vi "Autonomous Independent.vi"() -> ()   [LabVIEW 2013]
doc: "If AutoIDs match then TwoBall? is read from Dashboard, Else it is a control on the Front Panel\n\nINPUTS:\nTwoBall?\nState (Init)\nCollectorArmSpeed\nBrakeDistance\nSlowdownDistance\n\nSTATES:\n\nINIT: Clapper - In, SonicShifter Actuates to Low Gear, RollerPnuematic - Out, Servo - SetAngle (Indicator on Front Panel), IF TwoBall? == True: LowerArm ELSE CheckHotGoal\n\nCHECKHOTGOAL: Runs IsHotGoalDB and puts HotGoal? into Shift Register\n\nLOWERARM: Clapper - OUT, Wait = LowerArmTimeout / 2, RollerPneumatic - WAIT, Collector- LOWER\nWhen Collector has finished or after timeout from LowerArmTimeout and two other timers, Collector - STOP\nIF TwoBall? == TRUE then Collect ELSE Drive12ft\n\nPRECOLLECT: CollectorWrapper - PRECOLLECT\n\nDRIVEBACK: TankDrive -SETVALUE and DriveBackSpeed goes into both desired speeds, Wait - DriveBackWait, TankDrive - SETVALUE and 0 for both desired speeds\n\nCOLLECT: CollectWrapper - COLLECT\n\nSTOPCOLLECT: CollectWrapper - STOP\n\nLIFTARM: Collector - RAISE, Wait - LiftArmWait, Collector - STOP\n\nRAISESERVO: Servo - SETANGLE, Servo takes in RaiseServoAngle from Front Panel\n\nDRIVE12FT: Sonar - READVALUE, AutoDistance - LINEAR, Takes in Drive12ftDistance and distance from the Sonar and BrakeDistance and SlowdownDistance, TankDrive - LINEARDRIVE, Takes in both motor values from AutoDistance and MaxMotorChangeForward/Backward for Desired, TankDrive - LINEARDRIVE, Takes in 0 for Desired and MaxMotorChanges\n\nSHOOT12FT: IF not TwoBall? AND not HotGoal? then Wait - 5500 - ElapsedTime ELSE Pass, Wait - PreShootWait, ShooterWrapper - COLLECTORDOWN\n\nRAISEARM: Wait - PreRaiseArmWait, Collector - RAISE, Takes in CollectorArmSpeed, After Timeout from RaiseArmTimeout or Collector is done , Collector - STOP\n\nSHOOT3FT: Sonar - READVALUE, AutoDistance - LINEAR, Takes in Drive3ftDistance and output form Sonar and Brake/SlowdownDistance, TankDrive - SETVALUE, Takes in AutoDistance values for desired, Exits after AutoDistance is done or Drive3tfTimeout, TankDrive - SETVALUE, Takes in 0 for desired\n\nSHOOT3FT: ShooterWrapper - COLLECTORUP\n\nSTOP: Servo - SETANGLE, 0 for angle"
uses:
  AutoStates.ctl
  AutoMode.ctl
  HotGoalDetectType.ctl
  SingleSolenoidAction.ctl
  DoubleSolenoidAction.ctl
  ServoAction.ctl
  CollectorAction.ctl
  RollerAction.ctl
  TankDriveAction.ctl
  CollectorWrapAction.ctl
  SonarAction.ctl
  AutoAlignMode.ctl
  ShooterWrapperAction.ctl
  Robot Global Data.vi
panel:
  in  "PreScumbagWait":u32
  in  "HotGoalTypeDefault":T1
  out "KinectTriggered?":bool
  in  "EndInLowGear?":bool=TRUE
  in  "DriveBackWait":u32=1000
  in  "DriveBackSpeed":dbl=-1.0
  in  "PreCheckGoalWait":u32=260
  in  "BallSettleWait":u32=130
  in  "StartShootTime":u32=5000
  in  "StartInLowGear?":bool=TRUE
  in  "PreCollectWait":u32=400
  in  "AutoIDKey":i32=3061
  in  "DefaultMotorInput":dbl=1.0
  in  "DriveMinTime":u32=2000
  in  "RotateWait":u32=300
  in  "RotateMotorInput":dbl=0.7
  in  "DriveDistance":dbl=36.0 format="%#_13g"
  in  "DriveTimeout":u32=4000
  out "CheckGoalTimedOut?":bool
  in  "CheckHotGoalTimeout":u32=800
  in  "AutoDefaultMode":T2
  in  "ServoInitAngle":i32=140
  in  "RaiseServoAngle":i32=100
  in  "AccelBackward":dbl=0.1
  in  "PreRaiseArmWait":u32=500
  in  "AccelForward":dbl=0.1
  out "ElapsedTime":u32
  out "StateTime":u32
  out "CurrentState":T3
  out "RaiseArmTimedOut":bool
  out "Hot?":bool
  out "DriveTimeOut":bool
  out "LowerArmTimedOut":bool
  in  "RaiseArmTimeout":u32=800
  in  "SlowdownDistance":dbl=36.0 format="%#_13g"
  in  "BrakeDistance":dbl=12.0 format="%#_13g"
  in  "CollectorArmSpeed":dbl=1.0 format="%#_13g"
  in  "LiftArmWait":u32=200
  in  "PreDriveBackWait":u32
  in  "PreDriveBackSpeed":dbl
  in  "LowerArmTimeout":u32=800
  in  "error in":errorcluster
  out "error out":errorcluster
  # "SHOOT"
  # "SERVO"
  # "HOT GOAL"
  # "OUTPUT"
  # "ROTATE"
  # "GENERAL"
  # "DRIVE"
  # "RAISE/LOWER ARM"
  # "DEPRECATED"
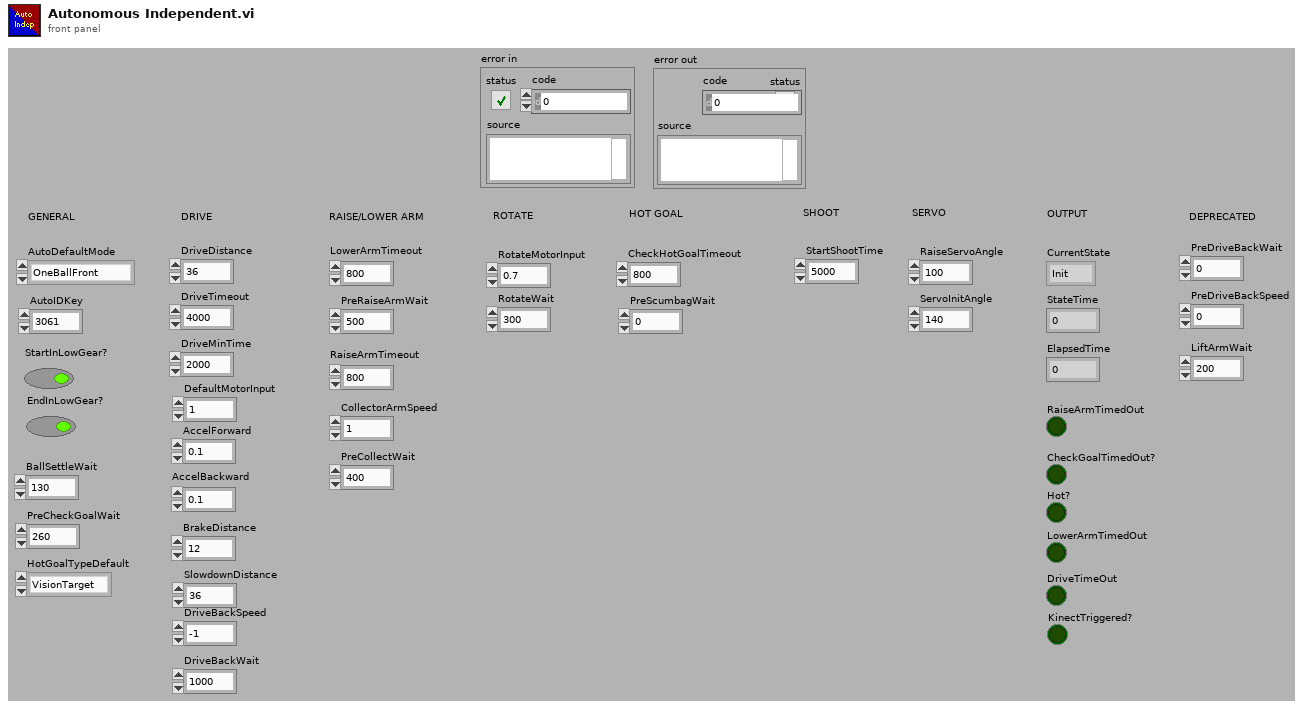
[diagram p1: front panel]
types:
  T1 = typedef "HotGoalDetectType.ctl" = enum16{"VisionTarget", "Kinect", "SoundDetect", "Webcam"}
  T2 = typedef "AutoMode.ctl" = enum16{"OneBallFront", "OneBallCollector", "TwoBallNormal", "TwoBallHot"}
  T3 = typedef "AutoStates.ctl" = enum16{"Init", "LowerArmCheckGoal", "DriveBack", "Collect", "StopCollect", "LiftArm", "RaiseServo", "Drive", "ShootCollectorUp", "RaiseArm", "ShootCollectorDown", "Rotate1", "Rotate2", "Stop"}
  T4 = typedef "SingleSolenoidAction.ctl" = enum16{"Init", "SetState", "Disable"}
  T5 = typedef "DoubleSolenoidAction.ctl" = enum16{"Init", "Middle", "In", "Out"}
  T6 = typedef "ServoAction.ctl" = enum16{"Init", "SetAngle", "GetAngle", "Lower", "Raise", "Disable"}
  T7 = typedef "CollectorAction.ctl" = enum16{"Init", "Raise", "Lower", "Stop", "GetStatus"}
  T8 = typedef "RollerAction.ctl" = enum16{"Init", "Off", "Forward", "Reverse"}
  T9 = typedef "TankDriveAction.ctl" = enum16{"Init", "LinearDrive", "SetValue", "Disable"}
  T10 = typedef "CollectorWrapAction.ctl" = enum16{"Stop", "PreCollect", "Collect"}
  T11 = typedef "AutoAlignMode.ctl" = enum16{"Fullspeed", "Linear"}
  T12 = typedef "SonarAction.ctl" = enum16{"Init", "ReadValue", "Disable"}
  T13 = typedef "ShooterWrapperAction.ctl" = enum16{"Init", "CollectorDown", "CollectorUp"}
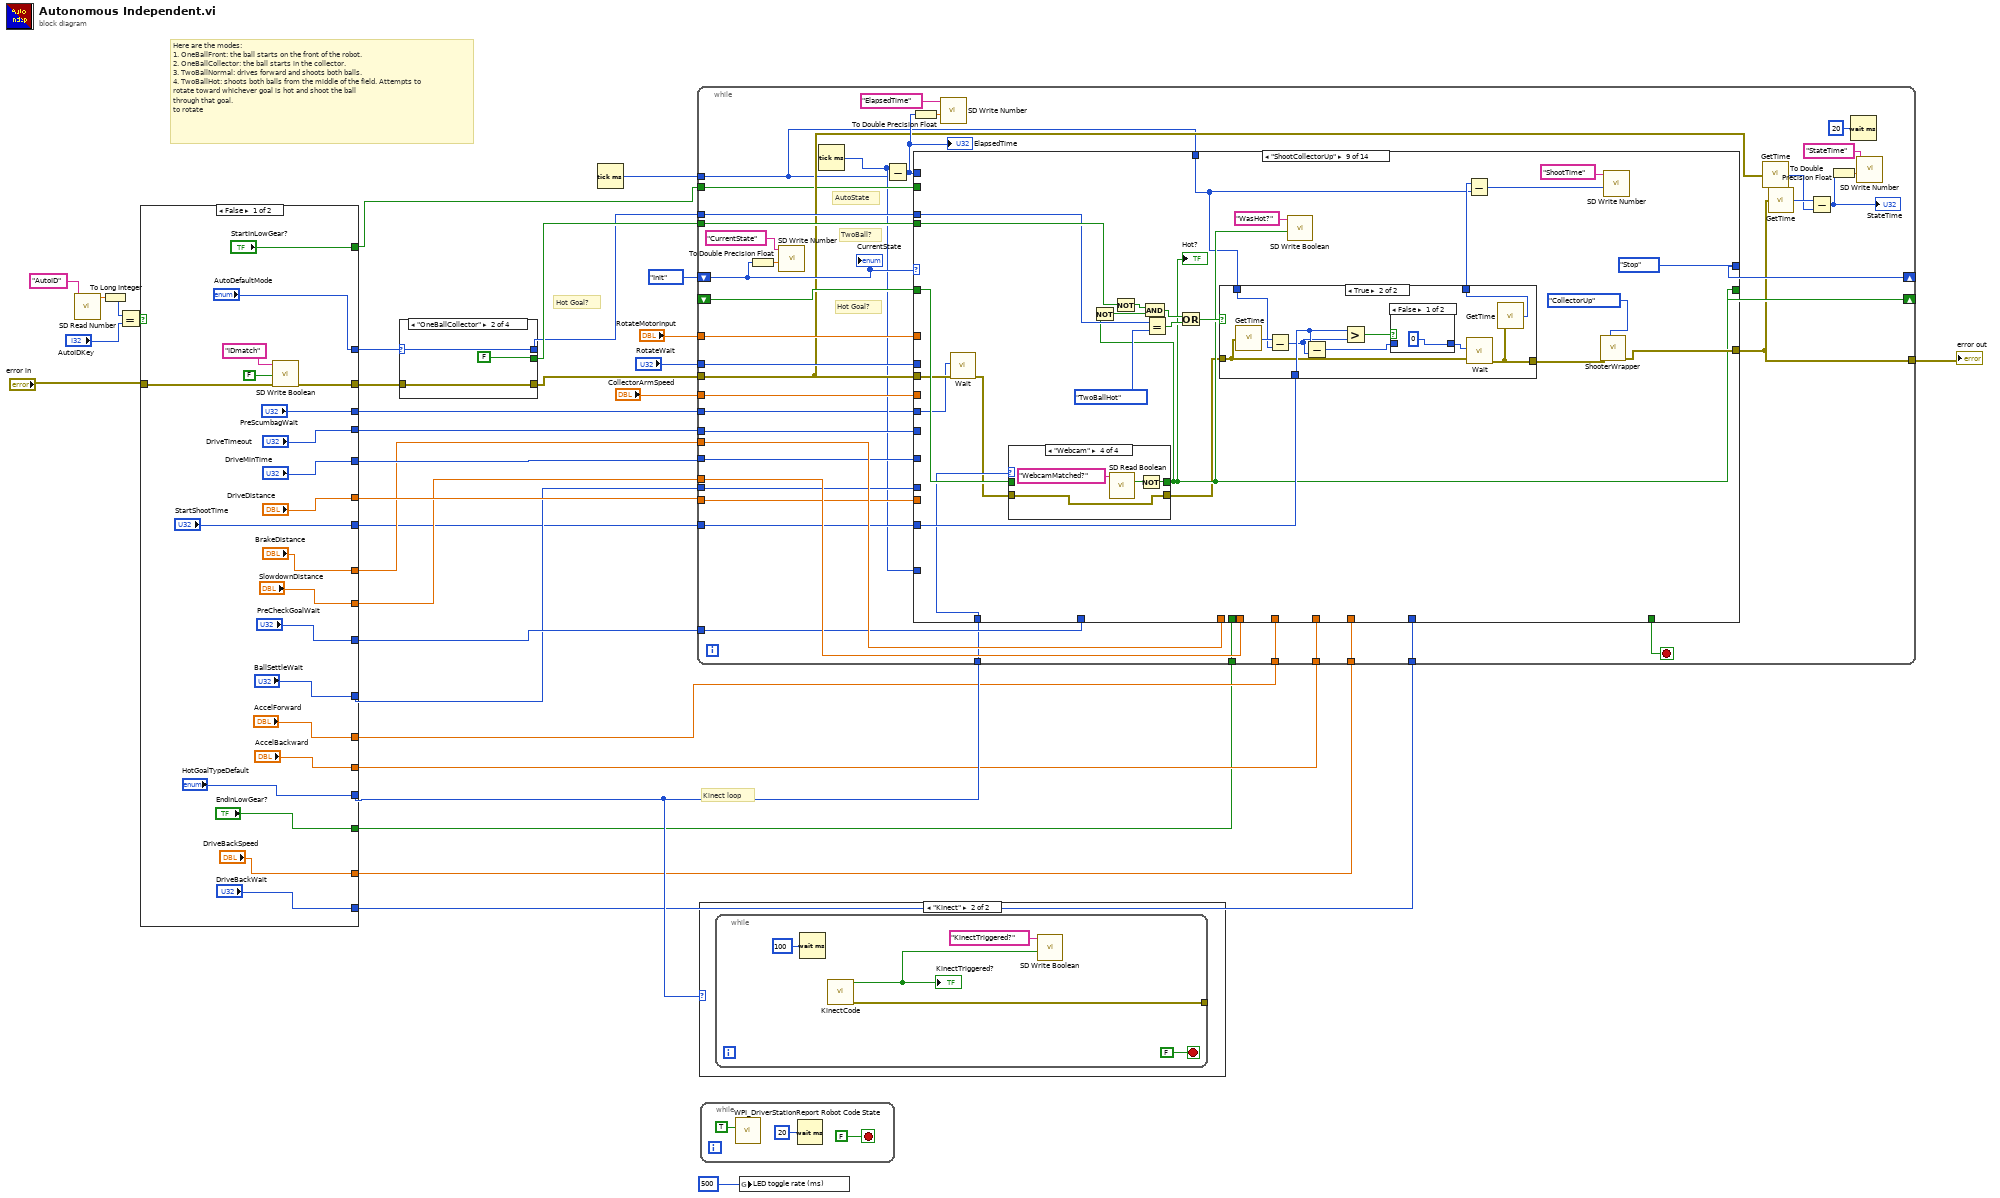
[diagram p0: block diagram]
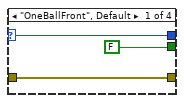
[diagram p3: hidden frame]
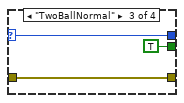
[diagram p4: hidden frame]
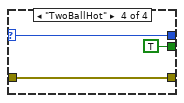
[diagram p5: hidden frame]
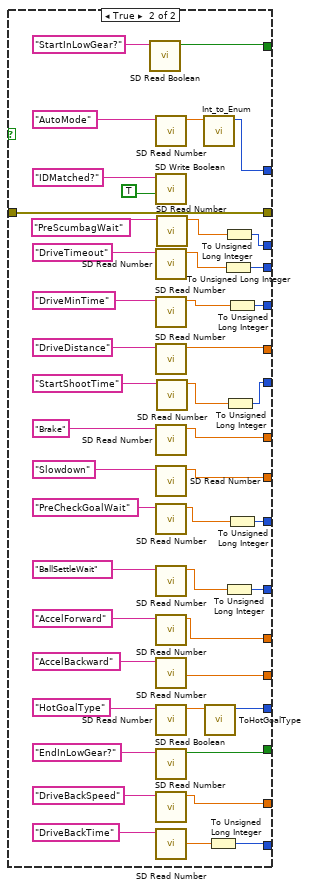
[diagram p6: hidden frame]
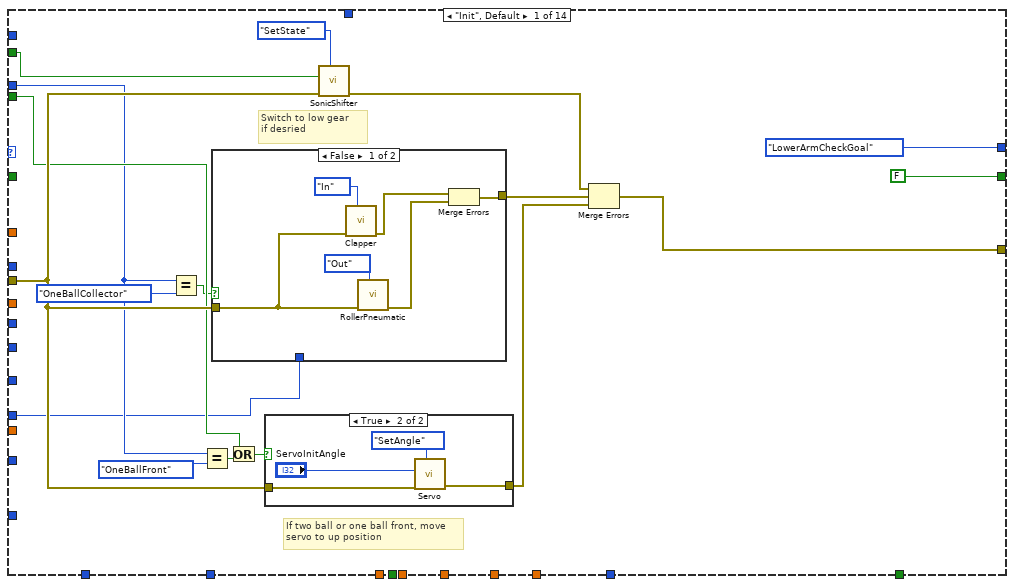
[diagram p7: hidden frame]
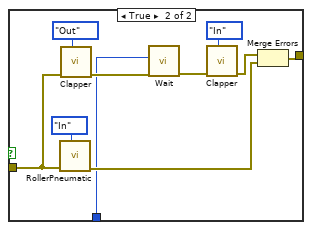
[diagram p8: hidden frame]
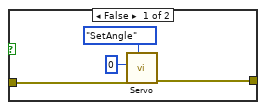
[diagram p9: hidden frame]
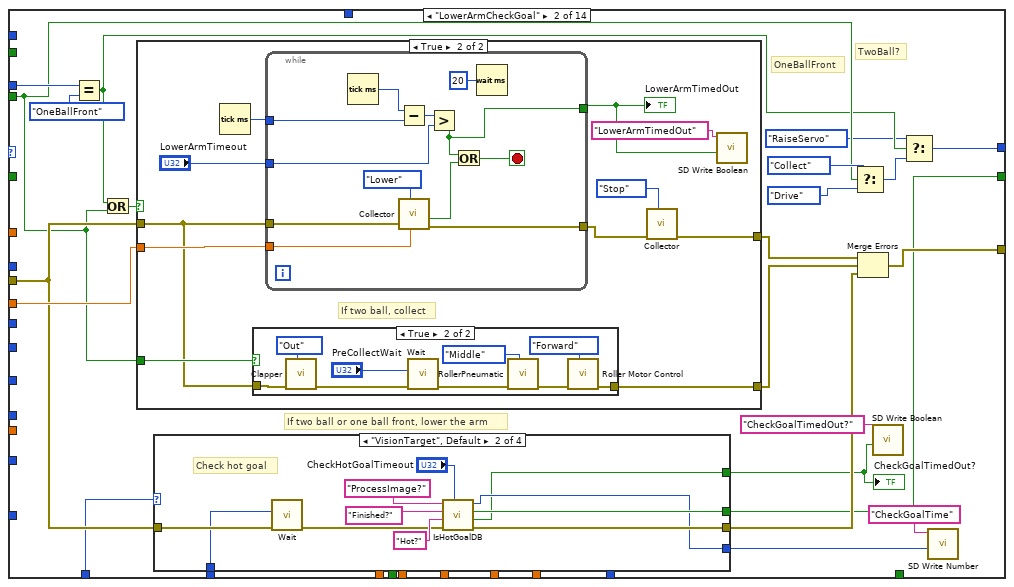
[diagram p10: hidden frame]
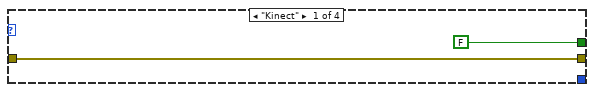
[diagram p11: hidden frame]
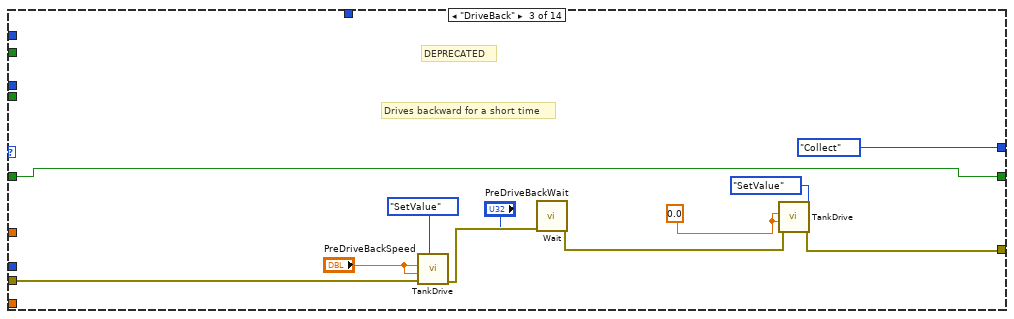
[diagram p16: hidden frame]
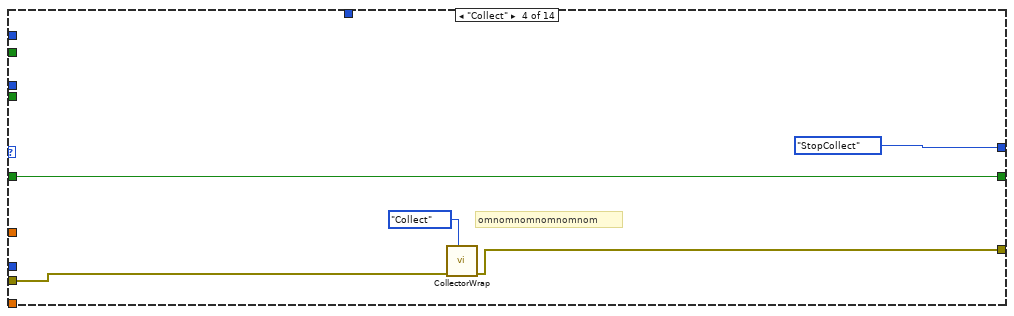
[diagram p17: hidden frame]
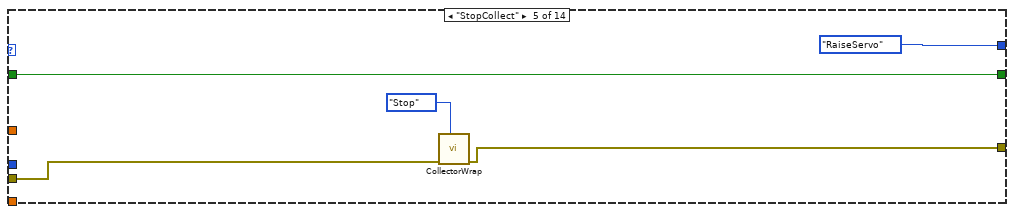
[diagram p18: hidden frame]
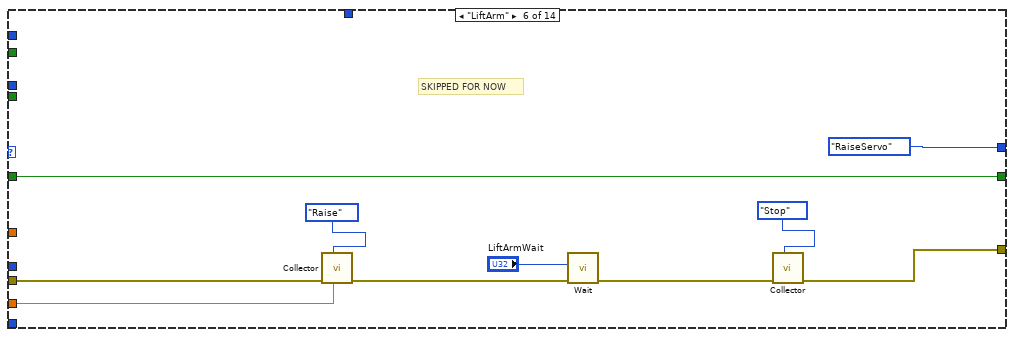
[diagram p19: hidden frame]
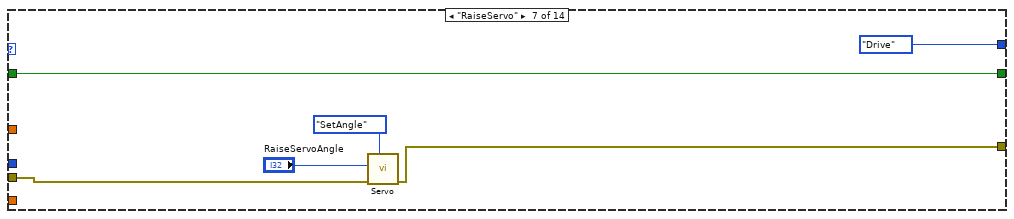
[diagram p20: hidden frame]
diagram:
  # "Kinect loop"
  # "Here are the modes:\n1. OneBallFront: the ball starts on the front of the robot.\n2. OneBallCollector: the ball starts in the collector.\n3. TwoBallNormal: drives forward and shoots both balls.\n4. TwoBallHot: shoots both balls from the middle of the field. Attempts to rotate toward whichever goal is hot and shoot the ball\nthrough that goal.\nto rotate"
  # "Hot Goal?"
  n1 = call <vilib>:"SD Read Number.vi"("Name"="AutoID") -> ("Numeric"=w33:dbl)  [unwired: 8 in, 2 out]
  n2 = To Long Integer(number=w33) -> (32bit integer=w19:i32)
  n3 = Equal?(x=w19, y="AutoIDKey") -> (x = y?=w28:bool)
  n4 = case shown="False" w28 {
    tunnel: "error in" -> [w54 w62]
    tunnel: [w53 w62] -> w24
    tunnel: ["AutoDefaultMode" w98] -> w26
    tunnel: ["DriveTimeout" w93] -> w14
    tunnel: ["DriveMinTime" w91] -> w15
    tunnel: ["DriveDistance" w89] -> w16
    tunnel: ["BrakeDistance" w87] -> w13
    tunnel: ["SlowdownDistance" w86] -> w12
    tunnel: ["PreCheckGoalWait" w83] -> w11
    tunnel: ["BallSettleWait" w80] -> w10
    tunnel: ["HotGoalTypeDefault" w76] -> w9
    tunnel: ["StartInLowGear?" w75] -> w8
    tunnel: ["AccelForward" w71] -> w7
    tunnel: ["AccelBackward" w70] -> w6
    tunnel: ["EndInLowGear?" w68] -> w5
    tunnel: ["DriveBackSpeed" w66] -> w4
    tunnel: ["DriveBackWait" w63] -> w3
    tunnel: ["StartShootTime" w59] -> w2
    tunnel: ["PreScumbagWait" w56] -> w1
    frame False {
      n5 = call <vilib>:"SD Write Boolean.vi"("error in"=w54, "Boolean"=FALSE, "Name"="IDmatch") -> ("error out"=w53:errorcluster)  [unwired: 7 in, 1 out]
    }
    frame True {
      n6 = call <vilib>:"SD Read Boolean.vi"("Name"="StartInLowGear?") -> ("Boolean"=w75:bool)  [unwired: 8 in, 2 out]
      n7 = call <vilib>:"SD Read Number.vi"("Name"="AutoMode") -> ("Numeric"=w99:dbl)  [unwired: 8 in, 2 out]
      n8 = call <vilib>:"SD Write Boolean.vi"("Boolean"=TRUE, "Name"="IDMatched?") -> ()  [unwired: 8 in, 2 out]
      n9 = call <vilib>:"SD Read Number.vi"("Name"="DriveTimeout") -> ("Numeric"=w92:dbl)  [unwired: 8 in, 2 out]
      n10 = call <vilib>:"SD Read Number.vi"("Name"="DriveMinTime") -> ("Numeric"=w90:dbl)  [unwired: 8 in, 2 out]
      n11 = call <vilib>:"SD Read Number.vi"("Name"="DriveDistance") -> ("Numeric"=w89:dbl)  [unwired: 8 in, 2 out]
      n12 = call <vilib>:"SD Read Number.vi"("Name"="Brake") -> ("Numeric"=w87:dbl)  [unwired: 8 in, 2 out]
      n13 = call <vilib>:"SD Read Number.vi"("Name"="Slowdown") -> ("Numeric"=w86:dbl)  [unwired: 8 in, 2 out]
      n14 = call <vilib>:"SD Read Number.vi"("Name"="PreCheckGoalWait") -> ("Numeric"=w82:dbl)  [unwired: 8 in, 2 out]
      n15 = call <vilib>:"SD Read Number.vi"("Name"="BallSettleWait") -> ("Numeric"=w79:dbl)  [unwired: 8 in, 2 out]
      n16 = call <vilib>:"SD Read Number.vi"("Name"="AccelForward") -> ("Numeric"=w71:dbl)  [unwired: 8 in, 2 out]
      n17 = call <vilib>:"SD Read Number.vi"("Name"="AccelBackward") -> ("Numeric"=w70:dbl)  [unwired: 8 in, 2 out]
      n18 = call <vilib>:"SD Read Number.vi"("Name"="HotGoalType") -> ("Numeric"=w77:dbl)  [unwired: 8 in, 2 out]
      n19 = call <vilib>:"SD Read Boolean.vi"("Name"="EndInLowGear?") -> ("Boolean"=w68:bool)  [unwired: 8 in, 2 out]
      n20 = call <vilib>:"SD Read Number.vi"("Name"="DriveBackSpeed") -> ("Numeric"=w66:dbl)  [unwired: 8 in, 2 out]
      n21 = call <vilib>:"SD Read Number.vi"("Name"="DriveBackTime") -> ("Numeric"=w65:dbl)  [unwired: 8 in, 2 out]
      n22 = call <vilib>:"SD Read Number.vi"("Name"="PreScumbagWait") -> ("Numeric"=w58:dbl)  [unwired: 8 in, 2 out]
      n23 = call <vilib>:"SD Read Number.vi"("Name"="StartShootTime") -> ("Numeric"=w61:dbl)  [unwired: 8 in, 2 out]
      n24 = call "Int_to_Enum.vi"("IntIn"=w99) -> ("EnumOut"=w98:T2)  [unwired: 10 in]
      n25 = call "ToHotGoalType.vi"("IntIn"=w77) -> ("EnumOut"=w76:T1)  [unwired: 10 in]
      n26 = To Unsigned Long Integer(number=w65) -> (unsigned 32bit integer=w63:u32)
      n27 = To Unsigned Long Integer(number=w92) -> (unsigned 32bit integer=w93:u32)
      n28 = To Unsigned Long Integer(number=w58) -> (unsigned 32bit integer=w56:u32)
      n29 = To Unsigned Long Integer(number=w79) -> (unsigned 32bit integer=w80:u32)
      n30 = To Unsigned Long Integer(number=w61) -> (unsigned 32bit integer=w59:u32)
      n31 = To Unsigned Long Integer(number=w90) -> (unsigned 32bit integer=w91:u32)
      n32 = To Unsigned Long Integer(number=w82) -> (unsigned 32bit integer=w83:u32)
    }
  }
  n33 = case shown="\"OneBallCollector\"" w26 {
    selector: w26 -> [w102 w105 w108 w111]
    tunnel: [FALSE FALSE TRUE TRUE] -> w25
    tunnel: w24 -> [w103 w106 w109 w112]
    tunnel: [w103 w106 w109 w112] -> w23
    tunnel: [w102 w105 w108 w111] -> w22
    frame "OneBallFront", Default {
    }
    frame "OneBallCollector" {
    }
    frame "TwoBallNormal" {
    }
    frame "TwoBallHot" {
    }
  }
  n34 = Tick Count (ms)() -> (millisecond timer value=w29:u32)
  n35 = while {
    shift-right: [w152] -> _
    shift-left: AutoStates."Init" ("Enum") -> [w134]
    shift-right: [w154] -> _
    shift-left: _ -> [w153]
    tunnel: w25 -> [w151]
    tunnel: "CollectorArmSpeed" -> [w149]
    tunnel: w13 -> [w147]
    tunnel: w12 -> [w148]
    tunnel: w29 -> [w114]
    tunnel: w23 -> [w131]
    tunnel: [w132] -> w34
    tunnel: w22 -> [w144]
    tunnel: "RotateMotorInput" -> [w143]
    tunnel: "RotateWait" -> [w142]
    tunnel: w2 -> [w129]
    tunnel: w16 -> [w128]
    tunnel: w15 -> [w127]
    tunnel: w14 -> [w126]
    tunnel: w11 -> [w125]
    tunnel: w10 -> [w124]
    tunnel: w9 -> [w123]
    tunnel: w8 -> [w122]
    tunnel: w7 -> [w121]
    tunnel: w6 -> [w120]
    tunnel: w5 -> [w118]
    tunnel: w4 -> [w117]
    tunnel: w3 -> [w116]
    tunnel: w1 -> [w115]
    stop <- w146 stop-if-true
    # "AutoState"
    # "TwoBall?"
    # "Hot Goal?"
    n36 = To Double Precision Float(number=w134) -> (double precision float=w135:dbl)
    n37 = call <vilib>:"SD Write Number.vi"("Numeric"=w135, "Name"="CurrentState") -> ()  [unwired: 8 in, 2 out]
    n38 = Tick Count (ms)() -> (millisecond timer value=w119:u32)
    n39 = Subtract(x=w119, y=w114) -> (x-y=w137:u32)
    "ElapsedTime" <- w137
    n40 = To Double Precision Float(number=w137) -> (double precision float=w136:dbl)
    n41 = case shown="\"ShootCollectorUp\"" w134 {
      selector: w134 -> [_ _ _ _ _ _ _ _ _ _ _ _ _ w543]
      tunnel: w131 -> [w166 w216 w278 w283 w288 w293 w303 w335 w392 w457 w478 w501 w517 w544]
      tunnel: [w170 w215 w271 w282 w287 w292 w302 w332 w411 w455 w483 w496 w516 w531] -> w132
      tunnel: [FALSE ("Hot?") w202 w276 w280 w285 w291 w304 w324 w396 w456 w473 w499 w510 w545] -> w154
      tunnel: w153 -> [_ _ w276 w280 w285 w291 w304 w324 w399 w456 w473 w499 w510 w545]
      tunnel: [AutoStates."LowerArmCheckGoal" ("Enum") w203 AutoStates."Collect" ("Enum") AutoStates."StopCollect" ("Enum") AutoStates."RaiseServo" ("Enum") AutoStates."RaiseServo" ("Enum") AutoStates."Drive" ("Enum") w322 AutoStates."Stop" ("Enum") w441 AutoStates."RaiseArm" ("Enum") AutoStates."ShootCollectorDown" ("Enum") AutoStates."ShootCollectorUp" ("Enum") w543] -> w152
      tunnel: w151 -> [w162 w208 _ _ _ _ _ _ w408 w450 w476 _ _ _]
      tunnel: w149 -> [_ w217 _ _ _ w290 _ _ _ w458 _ _ _ _]
      tunnel: w148 -> [_ _ _ _ _ _ _ w334 _ _ _ _ _ _]
      tunnel: w147 -> [_ _ _ _ _ _ _ w333 _ _ _ _ _ _]
      tunnel: w137 -> [_ _ _ _ _ _ _ _ _ _ w475 _ _ _]
      tunnel: [_ _ _ _ _ _ _ _ _ _ _ _ _ TRUE] -> w146
      tunnel: w144 -> [w158 w209 _ _ _ _ _ w320 w402 w446 _ _ _ _]
      tunnel: w143 -> [_ _ _ _ _ _ _ _ _ _ _ w506 w519 _]
      tunnel: w142 -> [_ _ _ _ _ _ _ _ _ _ _ w498 w518 _]
      tunnel: w129 -> [_ _ _ _ _ _ _ _ w400 _ w472 _ _ _]
      tunnel: w128 -> [_ _ _ _ _ _ _ w314 _ _ _ _ _ _]
      tunnel: w127 -> [_ _ _ _ _ _ _ w313 _ _ _ _ _ _]
      tunnel: w126 -> [_ _ _ _ _ _ _ w312 _ _ _ _ _ _]
      tunnel: w125 -> [_ w201 _ _ _ _ _ _ _ _ _ _ _ _]
      tunnel: w124 -> [w156 _ _ _ _ _ _ _ _ _ _ _ _ _]
      tunnel: w123 -> [_ w200 _ _ _ _ _ _ w398 _ _ _ _ _]
      tunnel: w122 -> [w155 _ _ _ _ _ _ _ _ _ _ _ _ _]
      tunnel: w121 -> [_ _ _ _ _ _ _ w311 _ _ _ _ _ _]
      tunnel: w120 -> [_ _ _ _ _ _ _ w310 _ _ _ _ _ _]
      tunnel: w119 -> [_ _ _ _ _ _ _ w306 _ _ _ _ _ _]
      tunnel: w118 -> [_ _ _ _ _ _ _ _ _ _ _ _ _ w530]
      tunnel: w117 -> [_ _ _ _ _ _ _ _ _ _ _ _ _ w529]
      tunnel: w116 -> [_ _ _ _ _ _ _ _ _ _ _ _ _ w528]
      tunnel: w115 -> [_ _ _ _ _ _ _ _ w389 _ _ _ _ _]
      tunnel: w114 -> [_ _ _ _ _ _ _ _ w387 _ _ _ _ _]
      frame "Init", Default {
        # "If two ball or one ball front, move\nservo to up position"
        # "Switch to low gear\nif desried"
        n42 = Equal?(x=w158, y=AutoMode."OneBallCollector") -> (x = y?=w157:bool)
        n43 = Equal?(x=w158, y=AutoMode."OneBallFront") -> (x = y?=w161:bool)
        n44 = case shown="False" w157 {
          tunnel: [w175 w180] -> w171
          tunnel: w166 -> [w172 w185]
          tunnel: w156 -> [_ w178]
          frame False {
            n45 = call "Clapper.vi"("State"=DoubleSolenoidAction."In", "Error in"=w172) -> ("Error out"=w174:errorcluster)  [unwired: 9 in]
            n46 = call "RollerPneumatic.vi"("State"=DoubleSolenoidAction."Out", "Error in"=w172) -> ("Error out"=w173:errorcluster)  [unwired: 9 in]
            n47 = Merge Errors(w174, w173) -> (w175:errorcluster)
          }
          frame True {
            n48 = call "RollerPneumatic.vi"("State"=DoubleSolenoidAction."In", "Error in"=w185) -> ("Error out"=w181:errorcluster)  [unwired: 9 in]
            n49 = call "Clapper.vi"("State"=DoubleSolenoidAction."Out", "Error in"=w185) -> ("Error out"=w184:errorcluster)  [unwired: 9 in]
            n50 = call "Wait.vi"("error in"=w184, "milliseconds to wait"=w178) -> ("error out"=w183:errorcluster)  [unwired: 9 in]
            n51 = call "Clapper.vi"("State"=DoubleSolenoidAction."In", "Error in"=w183) -> ("Error out"=w182:errorcluster)  [unwired: 9 in]
            n52 = Merge Errors(w182, w181) -> (w180:errorcluster)
          }
        }
        n53 = Or(x=w162, y=w161) -> (x .or. y?=w163:bool)
        n54 = case shown="True" w163 {
          tunnel: w166 -> [w190 w195]
          tunnel: [w189 w194] -> w168
          frame False {
            n55 = call "Servo.vi"("Action"=ServoAction."SetAngle", "error in (no error)"=w190, "Angle (deg)"=0) -> ("error out"=w189:errorcluster)  [unwired: 7 in, 1 out]
          }
          frame True {
            n56 = call "Servo.vi"("Action"=ServoAction."SetAngle", "error in (no error)"=w195, "Angle (deg)"="ServoInitAngle") -> ("error out"=w194:errorcluster)  [unwired: 7 in, 1 out]
          }
        }
        n57 = call "SonicShifter.vi"("Action"=SingleSolenoidAction."SetState", "error in (no error)"=w166, "Actuate?"=w155) -> ("error out"=w167:errorcluster)  [unwired: 8 in]
        n58 = Merge Errors(w167, w171, w168) -> (w170:errorcluster)
      }
      frame "LowerArmCheckGoal" {
        # "If two ball or one ball front, lower the arm"
        # "OneBallFront"
        # "TwoBall?"
        n59 = Equal?(x=w209, y=AutoMode."OneBallFront") -> (x = y?=w206:bool)
        n60 = Or(x=w206, y=w208) -> (x .or. y?=w211:bool)
        n61 = case shown="True" w211 {
          tunnel: w217 -> [_ w244]
          tunnel: [w234 w243] -> w207
          tunnel: w216 -> [w234 w237]
          tunnel: [w234 w239] -> w212
          tunnel: w208 -> [_ w238]
          frame False {
          }
          frame True {
            # "If two ball, collect"
            n62 = Tick Count (ms)() -> (millisecond timer value=w245:u32)
            n63 = case shown="True" w238 {
              tunnel: [w246 w249] -> w239
              tunnel: w237 -> [w246 w250]
              frame False {
              }
              frame True {
                n64 = call "Clapper.vi"("State"=DoubleSolenoidAction."Out", "Error in"=w250) -> ("Error out"=w254:errorcluster)  [unwired: 9 in]
                n65 = call "Wait.vi"("error in"=w254, "milliseconds to wait"="PreCollectWait") -> ("error out"=w252:errorcluster)  [unwired: 9 in]
                n66 = call "RollerPneumatic.vi"("State"=DoubleSolenoidAction."Middle", "Error in"=w252) -> ("Error out"=w255:errorcluster)  [unwired: 9 in]
                n67 = call "Roller Motor Control.vi"("Action"=RollerAction."Forward", "Error in"=w255) -> ("Error out"=w249:errorcluster)  [unwired: 9 in]
              }
            }
            n68 = while {
              tunnel: w237 -> [w256]
              tunnel: [w267] -> w240
              tunnel: w245 -> [w260]
              tunnel: w244 -> [w259]
              tunnel: [w258] -> w236
              tunnel: "LowerArmTimeout" -> [w257]
              stop <- w262 stop-if-true
              n69 = Tick Count (ms)() -> (millisecond timer value=w264:u32)
              n70 = Subtract(x=w264, y=w260) -> (x-y=w265:u32)
              n71 = call "Collector.vi"("MotorSpeed"=w259, "Action"=CollectorAction."Lower", "Error in"=w256) -> ("Error out"=w267:errorcluster, "Lower Triggered?"=w261:bool)  [unwired: 6 in, 1 out]
              n72 = Greater?(x=w265, y=w257) -> (0:w258:bool)
              n73 = Or(x=w258, y=w261) -> (x .or. y?=w262:bool)
              n74 = Wait (ms)(milliseconds to wait=u32 20) -> ()  [unwired: 1 out]
            }
            "LowerArmTimedOut" <- w236
            n75 = call "Collector.vi"("Action"=CollectorAction."Stop", "Error in"=w240) -> ("Error out"=w243:errorcluster)  [unwired: 7 in, 2 out]
            n76 = call <vilib>:"SD Write Boolean.vi"("Boolean"=w236, "Name"="LowerArmTimedOut") -> ()  [unwired: 8 in, 2 out]
          }
        }
        n77 = case shown="\"VisionTarget\", Default" w200 {
          tunnel: w216 -> [w220 w227 w232 w233]
          tunnel: [w220 w226 w232 w233] -> w214
          tunnel: [FALSE ("Hot?") w223 _ _] -> w202
          tunnel: w201 -> [_ w224 _ _]
          tunnel: [_ w222 _ _] -> w197
          tunnel: [_ w221 _ _] -> w196
          frame "Kinect" {
          }
          frame "VisionTarget", Default {
            # "Check hot goal"
            n78 = call "Wait.vi"("error in"=w227, "milliseconds to wait"=w224) -> ("error out"=w225:errorcluster)  [unwired: 9 in]
            n79 = call "IsHotGoalDB.vi"("Timeout (ms)"="CheckHotGoalTimeout", "error in"=w225, "DBHot?"="Hot?", "DBFinished?"="Finished?", "DBStart"="ProcessImage?") -> ("error out"=w226:errorcluster, "TimedOut?"=w221:bool, "Hot?"=w223:bool, "ElapsedTime"=w222:u32)  [unwired: 3 in]
          }
          frame "SoundDetect" {
          }
          frame "Webcam" {
          }
        }
        "CheckGoalTimedOut?" <- w196
        n80 = Select(t=AutoStates."Collect" ("Enum"), s=w208, f=AutoStates."Drive" ("Enum")) -> (s? t:f=w204:T3)
        n81 = Merge Errors(w207, w212, w214) -> (w215:errorcluster)
        n82 = call <vilib>:"SD Write Boolean.vi"("Boolean"=w196, "Name"="CheckGoalTimedOut?") -> ()  [unwired: 8 in, 2 out]
        n83 = Select(t=AutoStates."RaiseServo" ("Enum"), s=w206, f=w204) -> (s? t:f=w203:T3)
        n84 = call <vilib>:"SD Write Number.vi"("Numeric"=w197, "Name"="CheckGoalTime") -> ()  [unwired: 8 in, 2 out]
      }
      frame "DriveBack" {
        w269 = 0.0 ("LeftDesired")
        # "Drives backward for a short time"
        # "DEPRECATED"
        n85 = call "TankDrive.vi"("DriveAction"=TankDriveAction."SetValue", "error in (no error)"=w278, "RightDesired"="PreDriveBackSpeed", "LeftDesired"="PreDriveBackSpeed") -> ("error out"=w277:errorcluster)  [unwired: 6 in, 1 out]
        n86 = call "Wait.vi"("error in"=w277, "milliseconds to wait"="PreDriveBackWait") -> ("error out"=w272:errorcluster)  [unwired: 9 in]
        n87 = call "TankDrive.vi"("DriveAction"=TankDriveAction."SetValue", "error in (no error)"=w272, "RightDesired"=w269, "LeftDesired"=w269) -> ("error out"=w271:errorcluster)  [unwired: 6 in, 1 out]
      }
      frame "Collect" {
        # "omnomnomnomnomnom"
        n88 = call "CollectorWrap.vi"("Action"=CollectorWrapAction."Collect", "error in"=w283) -> ("error out"=w282:errorcluster)  [unwired: 9 in]
      }
      frame "StopCollect" {
        n89 = call "CollectorWrap.vi"("Action"=CollectorWrapAction."Stop", "error in"=w288) -> ("error out"=w287:errorcluster)  [unwired: 9 in]
      }
      frame "LiftArm" {
        # "SKIPPED FOR NOW"
        n90 = call "Collector.vi"("MotorSpeed"=w290, "Action"=CollectorAction."Raise" ("CollectorAction"), "Error in"=w293) -> ("Error out"=w294:errorcluster)  [unwired: 6 in, 2 out]
        n91 = call "Wait.vi"("error in"=w294, "milliseconds to wait"="LiftArmWait") -> ("error out"=w295:errorcluster)  [unwired: 9 in]
        n92 = call "Collector.vi"("Action"=CollectorAction."Stop" ("CollectorAction"), "Error in"=w295) -> ("Error out"=w292:errorcluster)  [unwired: 7 in, 2 out]
      }
      frame "RaiseServo" {
        n93 = call "Servo.vi"("Action"=ServoAction."SetAngle", "error in (no error)"=w303, "Angle (deg)"="RaiseServoAngle") -> ("error out"=w302:errorcluster)  [unwired: 7 in, 1 out]
      }
      frame "Drive" {
        n94 = Tick Count (ms)() -> (millisecond timer value=w336:u32)
        n95 = while {
          tunnel: w335 -> [w366]
          tunnel: [w370] -> w317
          tunnel: w336 -> [w371]
          tunnel: w334 -> [w368]
          tunnel: w333 -> [w369]
          tunnel: [w353] -> w316
          tunnel: w311 -> [w362]
          tunnel: w310 -> [w361]
          tunnel: w312 -> [w360]
          tunnel: w314 -> [w359]
          tunnel: w313 -> [w354]
          stop <- w351 stop-if-true
          n96 = call "Sonar.vi"("Action"=SonarAction."ReadValue", "error in (no error)"=w366) -> ("error out"=w363:errorcluster, "distance"=w365:dbl)  [unwired: 8 in]
          n97 = Tick Count (ms)() -> (millisecond timer value=w372:u32)
          n98 = Subtract(x=w372, y=w371) -> (x-y=w355:u32)
          n99 = Greater?(x=w355, y=w360) -> (0:w353:bool)
          n100 = Greater?(x=w355, y=w354) -> (0:w348:bool)
          n101 = Not(x=w348) -> (.not. x?=w347:bool)
          n102 = call "AutoDistance.vi"("Auto"=TRUE, "Mode"=AutoAlignMode."Linear", "Slowdown"=w368, "Brake"=w369, "DesiredDistance"=w359, "CurrentDistance"=w365) -> ("TankDriveRight"=w357:dbl, "TankDriveLeft"=w356:dbl, "Finished"=w349:bool)  [unwired: 3 in]
          n103 = Or(x=w353, y=w349) -> (x .or. y?=w352:bool)
          n104 = And(x=w349, y=w347) -> (x .and. y?=w350:bool)
          n105 = case shown="True" w350 {
            tunnel: [w379 w385] -> w370
            tunnel: w363 -> [w378 w384]
            tunnel: w362 -> [w374 w383]
            tunnel: w361 -> [w375 w382]
            tunnel: w357 -> [w376 _]
            tunnel: w356 -> [w377 _]
            frame False {
              n106 = call "TankDrive.vi"("MaxMotorChangeForward"=w374, "MaxMotorChangeBackwrad"=w375, "DriveAction"=TankDriveAction."LinearDrive", "error in (no error)"=w378, "RightDesired"=w376, "LeftDesired"=w377) -> ("error out"=w379:errorcluster)  [unwired: 4 in, 1 out]
            }
            frame True {
              n107 = call "TankDrive.vi"("MaxMotorChangeForward"=w383, "MaxMotorChangeBackwrad"=w382, "DriveAction"=TankDriveAction."LinearDrive", "error in (no error)"=w384, "RightDesired"="DefaultMotorInput", "LeftDesired"="DefaultMotorInput") -> ("error out"=w385:errorcluster)  [unwired: 4 in, 1 out]
            }
          }
          n108 = Select(t=w352, s=w348, f=FALSE) -> (s? t:f=w351:bool)
          n109 = Wait (ms)(milliseconds to wait=u32 20) -> ()  [unwired: 1 out]
        }
        "DriveTimeOut" <- w316
        n110 = call <vilib>:"SD Write Boolean.vi"("Boolean"=w316, "Name"="DriveTimeOut") -> ()  [unwired: 8 in, 2 out]
        n111 = while {
          tunnel: w317 -> [w345]
          tunnel: [w344] -> w332
          tunnel: w311 -> [w339]
          tunnel: w310 -> [w338]
          tunnel: [w337] -> w307
          stop <- w340 stop-if-true
          w343 = 0.0 ("LeftDesired")
          n112 = Wait (ms)(milliseconds to wait=u32 20) -> ()  [unwired: 1 out]
          n113 = call "TankDrive.vi"("MaxMotorChangeForward"=w339, "MaxMotorChangeBackwrad"=w338, "DriveAction"=TankDriveAction."LinearDrive", "error in (no error)"=w345, "RightDesired"=w343, "LeftDesired"=w343) -> ("error out"=w344:errorcluster, "InRange?"=w340:bool)  [unwired: 4 in]
          n114 = Tick Count (ms)() -> (millisecond timer value=w337:u32)
        }
        n115 = Equal?(x=w320, y=AutoMode."TwoBallNormal") -> (x = y?=w330:bool)
        n116 = Equal?(x=w320, y=AutoMode."OneBallFront") -> (x = y?=w329:bool)
        n117 = Or(x=w330, y=w329) -> (x .or. y?=w325:bool)
        n118 = Equal?(x=AutoMode."TwoBallHot" ("y"), y=w320) -> (x = y?=w319:bool)
        n119 = Subtract(x=w307, y=w306) -> (x-y=w308:u32)
        n120 = Select(t=AutoStates."ShootCollectorDown" ("Enum"), s=w325, f=AutoStates."ShootCollectorUp") -> (s? t:f=w323:T3)
        n121 = To Double Precision Float(number=w308) -> (double precision float=w309:dbl)
        n122 = Select(t=AutoStates."Rotate1" ("Enum"), s=w319, f=w323) -> (s? t:f=w322:T3)
        n123 = call <vilib>:"SD Write Number.vi"("Numeric"=w309, "Name"="DriveElapsedTime") -> ()  [unwired: 8 in, 2 out]
      }
      frame "ShootCollectorUp" {
        n124 = call "Wait.vi"("error in"=w392, "milliseconds to wait"=w389) -> ("error out"=w391:errorcluster)  [unwired: 9 in]
        n125 = case shown="\"Webcam\"" w398 {
          tunnel: w399 -> [w413 _ _ _]
          tunnel: [w413 w415 w418 w421] -> w396
          tunnel: w391 -> [w412 w414 w417 w424]
          tunnel: [w412 w414 w417 w424] -> w390
          frame "VisionTarget", Default {
          }
          frame "Kinect" {
            n126 = local read "KinectTriggered?"() -> (w416:bool)
            n127 = Not(x=w416) -> (.not. x?=w415:bool)
          }
          frame "SoundDetect" {
            n128 = call <vilib>:"SD Read Boolean.vi"("Name"="PitchDetected") -> ("Boolean"=w420:bool)  [unwired: 8 in, 2 out]
            n129 = Not(x=w420) -> (.not. x?=w418:bool)
          }
          frame "Webcam" {
            n130 = call <vilib>:"SD Read Boolean.vi"("Name"="WebcamMatched?") -> ("Boolean"=w423:bool)  [unwired: 8 in, 2 out]
            n131 = Not(x=w423) -> (.not. x?=w421:bool)
          }
        }
        "Hot?" <- w396
        n132 = Not(x=w396) -> (.not. x?=w407:bool)
        n133 = Not(x=w408) -> (.not. x?=w409:bool)
        n134 = And(x=w409, y=w407) -> (x .and. y?=w405:bool)
        n135 = Equal?(x=w402, y=AutoMode."TwoBallHot") -> (x = y?=w403:bool)
        n136 = Or(x=w405, y=w403) -> (x .or. y?=w404:bool)
        n137 = case shown="True" w404 {
          tunnel: w390 -> [w426 w430]
          tunnel: [w426 w432] -> w393
          tunnel: w400 -> [_ w434]
          tunnel: [w425 w431] -> w388
          tunnel: w387 -> [_ w428]
          frame False {
            n138 = call "GetTime.vi"("error in"=w426) -> ("Time"=w425:u32)
          }
          frame True {
            n139 = call "GetTime.vi"("error in"=w430) -> ("Time"=w429:u32)
            n140 = Subtract(x=w429, y=w428) -> (x-y=w427:u32)
            n141 = Subtract(x=w434, y=w427) -> (x-y=w435:u32)
            n142 = Greater?(x=w434, y=w427) -> (0:w436:bool)
            n143 = case shown="False" w436 {
              tunnel: [u32 0 w438] -> w433
              tunnel: w435 -> [_ w438]
              frame False {
              }
              frame True {
              }
            }
            n144 = call "Wait.vi"("error in"=w430, "milliseconds to wait"=w433) -> ("error out"=w432:errorcluster)  [unwired: 9 in]
            n145 = call "GetTime.vi"("error in"=w432) -> ("Time"=w431:u32)
          }
        }
        n146 = call <vilib>:"SD Write Boolean.vi"("Boolean"=w396, "Name"="WasHot?") -> ()  [unwired: 8 in, 2 out]
        n147 = Subtract(x=w388, y=w387) -> (x-y=w394:u32)
        n148 = call "ShooterWrapper.vi"("Action"=ShooterWrapperAction."CollectorUp", "error in"=w393) -> ("error out"=w411:errorcluster)  [unwired: 8 in]
        n149 = call <vilib>:"SD Write Number.vi"("Numeric"=w394, "Name"="ShootTime") -> ()  [unwired: 8 in, 2 out]
      }
      frame "RaiseArm" {
        # "Hot Goal?"
        # "TwoBall?"
        # "Give shooter\ntime to come back down"
        n150 = call "Wait.vi"("error in"=w457, "milliseconds to wait"="PreRaiseArmWait") -> ("error out"=w453:errorcluster)  [unwired: 9 in]
        n151 = Tick Count (ms)() -> (millisecond timer value=w459:u32)
        n152 = while {
          tunnel: w453 -> [w471]
          tunnel: [w470] -> w451
          tunnel: w459 -> [w463]
          tunnel: w458 -> [w462]
          tunnel: [w461] -> w440
          stop <- w464 stop-if-true
          n153 = Tick Count (ms)() -> (millisecond timer value=w466:u32)
          n154 = Subtract(x=w466, y=w463) -> (x-y=w467:u32)
          n155 = call "Collector.vi"("MotorSpeed"=w462, "Action"=CollectorAction."Raise", "Error in"=w471) -> ("Error out"=w470:errorcluster, "Upper Triggered?"=w460:bool)  [unwired: 6 in, 1 out]
          n156 = Greater?(x=w467, y="RaiseArmTimeout") -> (0:w461:bool)
          n157 = Wait (ms)(milliseconds to wait=u32 20) -> ()  [unwired: 1 out]
          n158 = Or(x=w461, y=w460) -> (x .or. y?=w464:bool)
        }
        "RaiseArmTimedOut" <- w440
        n159 = call "Collector.vi"("Action"=CollectorAction."Stop", "Error in"=w451) -> ("Error out"=w455:errorcluster)  [unwired: 7 in, 2 out]
        n160 = call <vilib>:"SD Write Boolean.vi"("Boolean"=w440, "Name"="RaiseArmTimedOut") -> ()  [unwired: 8 in, 2 out]
        n161 = Equal?(x=w446, y=AutoMode."TwoBallHot") -> (x = y?=w444:bool)
        n162 = Not(x=w450) -> (.not. x?=w449:bool)
        n163 = Select(t=AutoStates."Stop" ("Enum"), s=w449, f=AutoStates."ShootCollectorUp" ("Enum")) -> (s? t:f=w442:T3)
        n164 = Select(t=AutoStates."Rotate2" ("Enum"), s=w444, f=w442) -> (s? t:f=w441:T3)
      }
      frame "ShootCollectorDown" {
        # "AND"
        # "001\n111\n010\n100"
        n165 = Not(x=w476) -> (.not. x?=w480:bool)
        n166 = Not(x=w473) -> (.not. x?=w479:bool)
        n167 = And(x=w480, y=w479) -> (x .and. y?=w474:bool)
        n168 = case shown="True" w474 {
          tunnel: w478 -> [w484 w491]
          tunnel: [w484 w490] -> w477
          tunnel: w475 -> [_ w489]
          tunnel: w472 -> [_ w485]
          frame False {
          }
          frame True {
            n169 = Subtract(x=w485, y=w489) -> (x-y=w486:u32)
            n170 = Greater?(x=w485, y=w489) -> (0:w488:bool)
            n171 = case shown="False" w488 {
              tunnel: [u32 0 w493] -> w487
              tunnel: w486 -> [_ w493]
              frame False {
              }
              frame True {
              }
            }
            n172 = call "Wait.vi"("error in"=w491, "milliseconds to wait"=w487) -> ("error out"=w490:errorcluster)  [unwired: 9 in]
          }
        }
        n173 = call "ShooterWrapper.vi"("Action"=ShooterWrapperAction."CollectorDown", "error in"=w477) -> ("error out"=w483:errorcluster)  [unwired: 8 in]
      }
      frame "Rotate1" {
        w495 = 0.0
        # "ASSUME CAMERA POINTED LEFT"
        n174 = Select(t=1.0, s=w499, f=-1.0) -> (s? t:f=w508:dbl)
        n175 = Multiply(x=w508, y=w506) -> (x*y=w505:dbl)
        n176 = Negate(x=w505) -> (-x=w504:dbl)
        n177 = call "TankDrive.vi"("DriveAction"=TankDriveAction."SetValue", "error in (no error)"=w501, "RightDesired"=w505, "LeftDesired"=w504) -> ("error out"=w500:errorcluster)  [unwired: 6 in, 1 out]
        n178 = call "Wait.vi"("error in"=w500, "milliseconds to wait"=w498) -> ("error out"=w497:errorcluster)  [unwired: 9 in]
        n179 = call "TankDrive.vi"("DriveAction"=TankDriveAction."SetValue", "error in (no error)"=w497, "RightDesired"=w495, "LeftDesired"=w495) -> ("error out"=w496:errorcluster)  [unwired: 6 in, 1 out]
      }
      frame "Rotate2" {
        w521 = 0.0
        n180 = Select(t=1.0, s=w510, f=-1.0) -> (s? t:f=w526:dbl)
        n181 = Multiply(x=w526, y=w519) -> (x*y=w515:dbl)
        n182 = Negate(x=w515) -> (-x=w514:dbl)
        n183 = call "TankDrive.vi"("DriveAction"=TankDriveAction."SetValue", "error in (no error)"=w517, "RightDesired"=w514, "LeftDesired"=w515) -> ("error out"=w523:errorcluster)  [unwired: 6 in, 1 out]
        n184 = Multiply(x=u32 2, y=w518) -> (x*y=w513:u32)
        n185 = call "Wait.vi"("error in"=w523, "milliseconds to wait"=w513) -> ("error out"=w522:errorcluster)  [unwired: 9 in]
        n186 = call "TankDrive.vi"("DriveAction"=TankDriveAction."SetValue", "error in (no error)"=w522, "RightDesired"=w521, "LeftDesired"=w521) -> ("error out"=w516:errorcluster)  [unwired: 6 in, 1 out]
      }
      frame "Stop" {
        w535 = 0.0 ("LeftDesired")
        n187 = call "Servo.vi"("Action"=ServoAction."SetAngle", "error in (no error)"=w544, "Angle (deg)"=0) -> ("error out"=w533:errorcluster)  [unwired: 7 in, 1 out]
        n188 = call "SonicShifter.vi"("Action"=SingleSolenoidAction."SetState", "error in (no error)"=w533, "Actuate?"=w530) -> ("error out"=w532:errorcluster)  [unwired: 8 in]
        n189 = call "TankDrive.vi"("DriveAction"=TankDriveAction."SetValue", "error in (no error)"=w532, "RightDesired"=w529, "LeftDesired"=w529) -> ("error out"=w537:errorcluster)  [unwired: 6 in, 1 out]
        n190 = call "Wait.vi"("error in"=w537, "milliseconds to wait"=w528) -> ("error out"=w536:errorcluster)  [unwired: 9 in]
        n191 = call "TankDrive.vi"("DriveAction"=TankDriveAction."SetValue", "error in (no error)"=w536, "RightDesired"=w535, "LeftDesired"=w535) -> ("error out"=w531:errorcluster)  [unwired: 6 in, 1 out]
      }
    }
    n192 = call <vilib>:"SD Write Number.vi"("Numeric"=w136, "Name"="ElapsedTime") -> ()  [unwired: 8 in, 2 out]
    n193 = call "GetTime.vi"("error in"=w131) -> ("Time"=w130:u32)
    n194 = call "GetTime.vi"("error in"=w132) -> ("Time"=w145:u32)
    n195 = Subtract(x=w145, y=w130) -> (x-y=w141:u32)
    "StateTime" <- w141
    n196 = To Double Precision Float(number=w141) -> (double precision float=w139:dbl)
    n197 = Wait (ms)(milliseconds to wait=u32 20) -> ()  [unwired: 1 out]
    n198 = call <vilib>:"SD Write Number.vi"("Numeric"=w139, "Name"="StateTime") -> ()  [unwired: 8 in, 2 out]
    "CurrentState" <- w134
  }
  "error out" <- w34
  n199 = case shown="\"Kinect\"" w9 {
    frame "VisionTarget", Default {
    }
    frame "Kinect" {
      n200 = while {
        tunnel: [w548] -> _
        stop <- FALSE stop-if-true
        n201 = Wait (ms)(milliseconds to wait=u32 100) -> ()  [unwired: 1 out]
        n202 = call "KinectCode.vi"() -> ("error out"=w548:errorcluster, "HandsApart?"=w547:bool)  [unwired: 10 in]
        "KinectTriggered?" <- w547
        n203 = call <vilib>:"SD Write Boolean.vi"("Boolean"=w547, "Name"="KinectTriggered?") -> ()  [unwired: 8 in, 2 out]
      }
    }
  }
  n204 = while {
    stop <- FALSE stop-if-true
    n205 = call <vilib>:"WPI_DriverStationReport Robot Code State.vi"("Autonomous"=TRUE) -> ()  [unwired: 10 in, 1 out]
    n206 = Wait (ms)(milliseconds to wait=u32 20) -> ()  [unwired: 1 out]
  }
  n207 = global write "Robot Global Data.vi" "LED toggle rate (ms)"(u32 500 ("LED ms toggle rate")) -> ()
